vi "Read.vi"(8 "error in (no error)":errorcluster, 10 "BytesToRead":i32, 11 "TcpClient in":refnum<class "TcpClient.lvclass">) -> (0 "error out":errorcluster, 2 "Data":string, 3 "TcpClient out":refnum<class "TcpClient.lvclass">)   [LabVIEW 2021, in "TcpClient.lvlib" / "TcpClient.lvclass"]
uses:
  TcpClient.lvclass
  TcpClient.lvclass/TcpClient.ctl
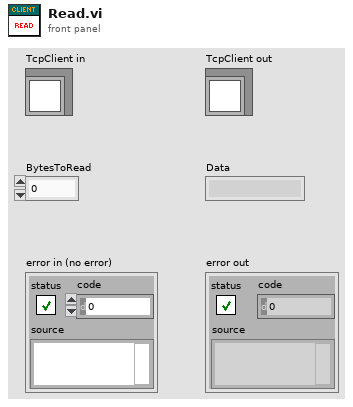
[diagram p1: front panel]
types:
  T1 = enum16{"Standard", "Buffered", "CRLF", "Immediate"}
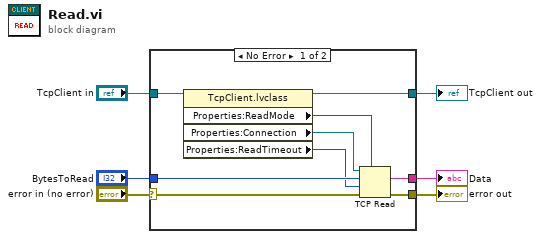
[diagram p0: block diagram]
diagram:
  n1 = case shown="No Error" "error in (no error)" {
    selector: "error in (no error)" -> [w15 w17]
    tunnel: [w14 w17] -> w5
    tunnel: [w10 w16] -> w3
    tunnel: "TcpClient in" -> [w13 w16]
    tunnel: "BytesToRead" -> [w12 _]
    tunnel: [w11 _] -> w1
    frame No Error {
      n2 = property class="TcpClient.lvclass"(reference=w13) -> (reference out=w10:refnum<class "TcpClient.lvclass">, "Properties:ReadMode"=w9:T1, "Properties:Connection"=w8:refnum<k5>, "Properties:ReadTimeout"=w7:i32)  [unwired: 1 in, 1 out]
      n3 = TCP Read(connection ID=w8, bytes to read=w12, error in (no error)=w15, 7:w9, 9:w7) -> (data out=w11:string, error out=w14:errorcluster)  [unwired: 1 out]
    }
    frame Error {
    }
  }
  "error out" <- w5
  "TcpClient out" <- w3
  "Data" <- w1
